vi "Check Key.vi"(8 "error in (no error)":errorcluster, 11 "[MV] Key Certify in":refnum<class "[MV] Key Certify.lvclass">) -> (0 "error out":errorcluster, 2 "valid?":bool, 3 "[MV] Key Certify out":refnum<class "[MV] Key Certify.lvclass">)   [LabVIEW 2020, in "[MV] Key Certify.lvlib" / "[MV] Key Certify.lvclass"]
uses:
  [MV] Key Certify.lvclass
  [MV] Key Certify.lvclass/[MV] Key Certify.ctl
  <vilib>/YU/YU-Encrypt/Base64/Base64.lvclass
  <vilib>/YU/YU-Encrypt/AES/AES.lvclass
  <vilib>/YU/YU-Encrypt/RSA/RSA.lvclass
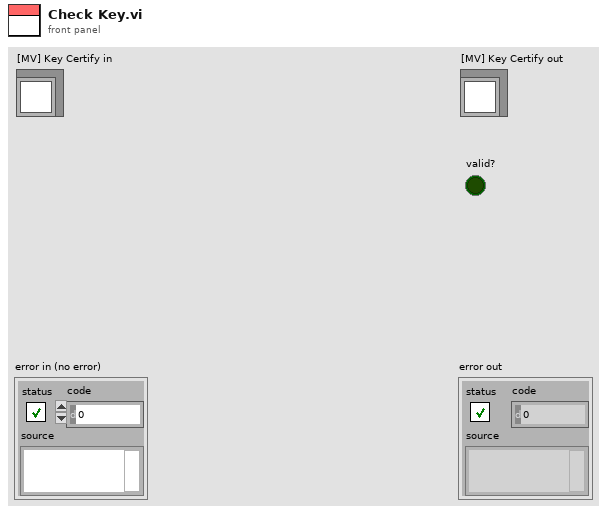
[diagram p1: front panel]
types:
  T1 = cluster{"machine_code":string, "sign_time":u64, "valid_days":i16}
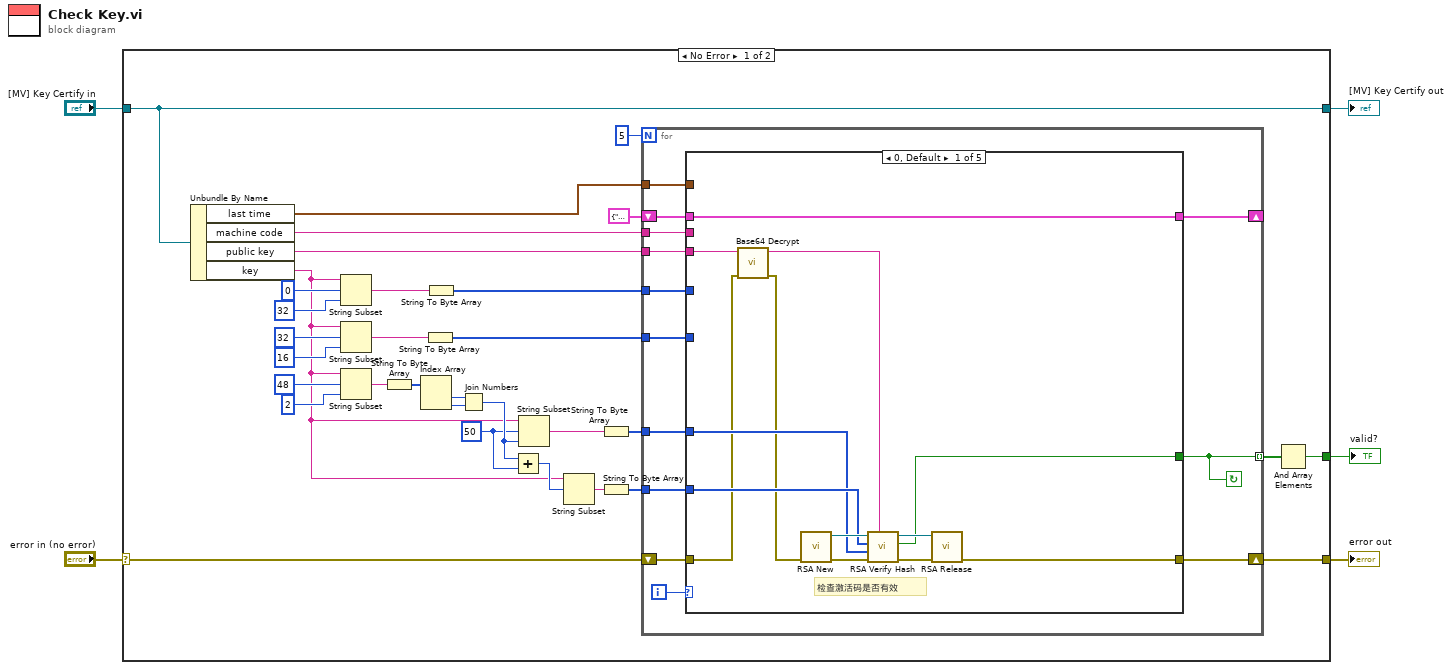
[diagram p0: block diagram]
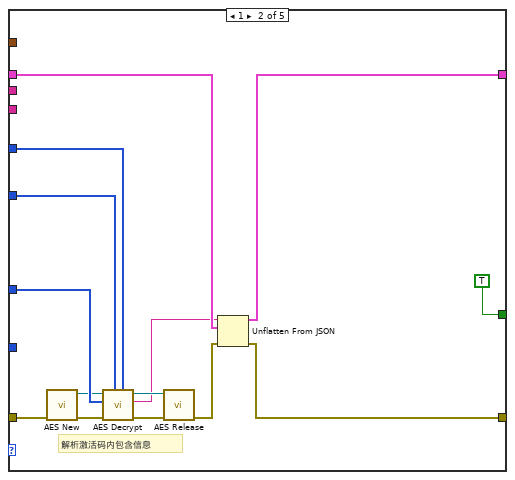
[diagram p2: hidden frame]
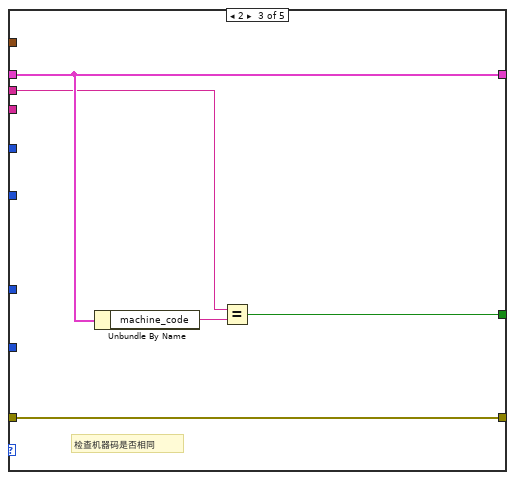
[diagram p3: hidden frame]
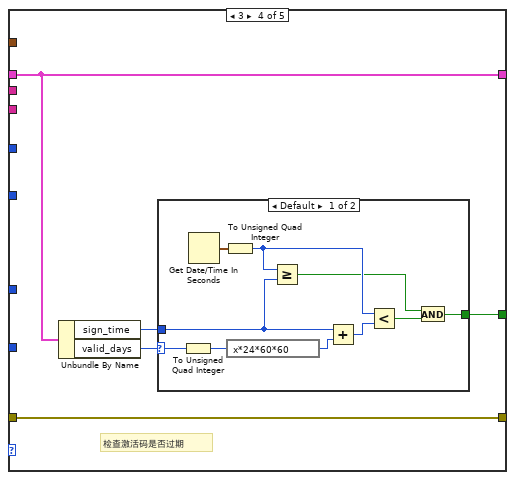
[diagram p4: hidden frame]
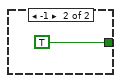
[diagram p5: hidden frame]
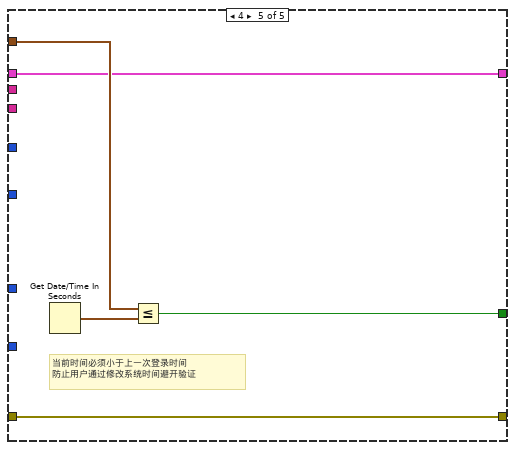
[diagram p6: hidden frame]
diagram:
  n1 = case shown="No Error" "error in (no error)" {
    selector: "error in (no error)" -> [w13 w105]
    tunnel: [w8 w105] -> w4
    tunnel: [w37 w104] -> w2
    tunnel: "[MV] Key Certify in" -> [w37 w104]
    tunnel: [w9 _] -> w1
    frame No Error {
      w25 = 50 ("offset (0)")
      n2 = Unbundle By Name(w37) -> ("last time"=w6:timestamp, "machine code"=w18:string, "public key"=w11:string, "key"=w19:string)
      n3 = String Subset(string=w19, offset (0)=0, length (rest)=32 ("length (rest)")) -> (substring=w21:string)
      n4 = String Subset(string=w19, offset (0)=32, length (rest)=16 ("length (rest)")) -> (substring=w20:string)
      n5 = String Subset(string=w19, offset (0)=48, length (rest)=2 ("length (rest)")) -> (substring=w30:string)
      n6 = String To Byte Array(string=w30) -> (unsigned byte array=w29:u8[])
      n7 = Index Array(array=w29) -> (element #1=w28:u8, element #2=w27:u8)  [unwired: 2 in]
      n8 = String To Byte Array(string=w20) -> (unsigned byte array=w16:u8[])
      n9 = String To Byte Array(string=w21) -> (unsigned byte array=w17:u8[])
      n10 = Join Numbers(hi=w28, lo=w27) -> ((hi.lo)=w26:u16)
      n11 = Add(x=w26, y=w25) -> (x+y=w24:i32)
      n12 = String Subset(string=w19, offset (0)=w25, length (rest)=w26) -> (substring=w22:string)
      n13 = String Subset(string=w19, offset (0)=w24) -> (substring=w23:string)  [unwired: 1 in]
      n14 = String To Byte Array(string=w22) -> (unsigned byte array=w15:u8[])
      n15 = String To Byte Array(string=w23) -> (unsigned byte array=w14:u8[])
      n16 = for {
        N: 5 -> [_]
        tunnel: w18 -> [w48]
        tunnel: w11 -> [w47]
        tunnel: w17 -> [w46]
        tunnel: w16 -> [w45]
        tunnel: w15 -> [w44]
        tunnel: w14 -> [w43]
        shift-right: [w40] -> w8
        shift-left: w13 -> [w49]
        shift-right: [w41] -> _
        shift-left: T1 {"machine_code"="", "sign_time"=0, "valid_days"=0} -> [w42]
        tunnel: [w39] -> w10 mode=indexing
        tunnel: w6 -> [w38]
        i -> [w50]
        stop <- w39 continue-if-true
        n17 = case shown="0, Default" w50 {
          tunnel: w49 -> [w52 w73 w78 w83 w99]
          tunnel: w48 -> [_ _ w81 _ _]
          tunnel: w47 -> [w54 _ _ _ _]
          tunnel: w46 -> [_ w68 _ _ _]
          tunnel: w45 -> [_ w69 _ _ _]
          tunnel: w44 -> [w55 w71 _ _ _]
          tunnel: w43 -> [w56 _ _ _ _]
          tunnel: w42 -> [w63 w77 w82 w86 w100]
          tunnel: [w63 w74 w82 w86 w100] -> w41
          tunnel: [w57 TRUE ("verify?") w80 w87 w101] -> w39
          tunnel: [w58 w75 w78 w83 w99] -> w40
          tunnel: w38 -> [_ _ _ _ w103]
          frame 0, Default {
            # "检查激活码是否有效"
            n18 = call <vilib>:"Base64 Decrypt.vi"("error in (no error)"=w52, "encrypted data"=w54) -> ("error out"=w51:errorcluster, "data"=w53:string)  [unwired: 8 in]
            n19 = call <vilib>:"RSA New.vi"("error in (no error)"=w51) -> ("error out"=w60:errorcluster, "RSA out"=w62:refnum<class "RSA.lvclass">)  [unwired: 9 in]
            n20 = call <vilib>:"RSA Verify Hash.vi"("public key"=w53, "error in (no error)"=w60, "data"=w55, "signed data"=w56, "RSA in"=w62) -> ("error out"=w59:errorcluster, "verify?"=w57:bool, "RSA out"=w61:refnum<class "RSA.lvclass">)  [unwired: 4 in]
            n21 = call <vilib>:"RSA Release.vi"("error in (no error)"=w59, "RSA in"=w61) -> ("error out"=w58:errorcluster)  [unwired: 9 in]
          }
          frame 1 {
            # "解析激活码内包含信息"
            n22 = call <vilib>:"AES New.vi"("error in (no error)"=w73) -> ("error out"=w72:errorcluster, "AES out"=w70:refnum<class "AES.lvclass">)  [unwired: 9 in]
            n23 = call <vilib>:"AES Decrypt.vi"("Key"=w68, "IV"=w69, "error in (no error)"=w72, "encrypted data"=w71, "AES in"=w70) -> ("error out"=w66:errorcluster, "data"=w65:string, "AES out"=w67:refnum<class "AES.lvclass">)  [unwired: 4 in]
            n24 = call <vilib>:"AES Release.vi"("error in (no error)"=w66, "AES in"=w67) -> ("error out"=w76:errorcluster)  [unwired: 9 in]
            n25 = Unflatten From JSON(JSON string=w65, type and defaults=w77, error in (no error)=w76) -> (value=w74:T1, error out=w75:errorcluster)  [unwired: 4 in]
          }
          frame 2 {
            # "检查机器码是否相同"
            n26 = Unbundle By Name(w82) -> ("machine_code"=w79:string)
            n27 = Equal?(x=w81, y=w79) -> (x = y?=w80:bool)
          }
          frame 3 {
            # "检查激活码是否过期"
            n28 = Unbundle By Name(w86) -> ("sign_time"=w85:u64, "valid_days"=w84:i16)
            n29 = case shown="Default" w84 {
              selector: w84 -> [w94 _]
              tunnel: w85 -> [w92 _]
              tunnel: [w89 TRUE] -> w87
              frame Default {
                n30 = To Unsigned Quad Integer(1:w94) -> (0:w93:u64)
                n31 = Get Date/Time In Seconds() -> (seconds since 1Jan1904=w96:timestamp)
                n32 = To Unsigned Quad Integer(1:w96) -> (0:w91:u64)
                n33 = expression code="x*24*60*60"(w93) -> (w97:u64)
                n34 = Greater Or Equal?(x=w91, y=w92) -> (x >= y?=w88:bool)
                n35 = Add(x=w92, y=w97) -> (x+y=w95:u64)
                n36 = Less?(x=w91, y=w95) -> (x < y?=w90:bool)
                n37 = And(x=w88, y=w90) -> (x .and. y?=w89:bool)
              }
              frame -1 {
              }
            }
          }
          frame 4 {
            # "当前时间必须小于上一次登录时间\n防止用户通过修改系统时间避开验证"
            n38 = Get Date/Time In Seconds() -> (seconds since 1Jan1904=w102:timestamp)
            n39 = Less Or Equal?(x=w103, y=w102) -> (x <= y?=w101:bool)
          }
        }
      }
      n40 = And Array Elements(Boolean array=w10) -> (logical AND=w9:bool)
    }
    frame Error {
    }
  }
  "error out" <- w4
  "[MV] Key Certify out" <- w2
  "valid?" <- w1
